vi "Ctor.vi"(7 "Dev Team":refnum<class "Team.lvclass">, 8 "error in (no error)":errorcluster) -> (0 "error out":errorcluster, 3 "SB App out":refnum<class "SB App.lvclass">)   [LabVIEW 2020, in "SB App.lvlib" / "SB App.lvclass"]
uses:
  SB App.lvclass
  SquareBattle/Team/Team.lvclass
  SB App.lvclass/SB App.ctl
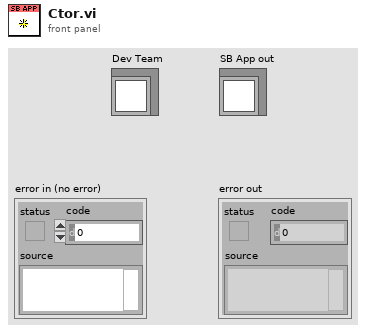
[diagram p1: front panel]
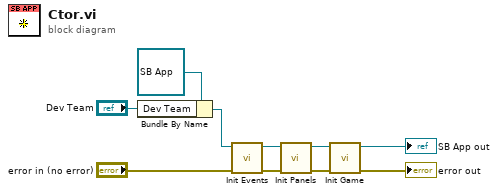
[diagram p0: block diagram]
diagram:
  n1 = Bundle By Name(cluster=refnum<class "SB App.lvclass"> refnum ("SB App in"), "Dev Team"="Dev Team") -> (w2:refnum<class "SB App.lvclass">)
  n2 = call "Init Events.vi"("error in (no error)"="error in (no error)", "SB App in"=w2) -> ("error out"=w7:errorcluster, "SB App out"=w8:refnum<class "SB App.lvclass">)  [unwired: 8 in]
  n3 = call "Init Panels.vi"("error in (no error)"=w7, "SB App in"=w8) -> ("error out"=w5:errorcluster, "SB App out"=w6:refnum<class "SB App.lvclass">)  [unwired: 8 in]
  n4 = call "Init Game.vi"("error in (no error)"=w5, "SB App in"=w6) -> ("error out"=→"error out":errorcluster, "SB App out"=→"SB App out":refnum<class "SB App.lvclass">)  [unwired: 8 in]
